vi "myRIO_BRig_Host_comm_hostRoot.vi"() -> (2 "output_hostRoot":string="C:\\BehaviorRig")   [LabVIEW 2014]
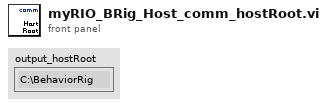
[diagram p1: front panel]
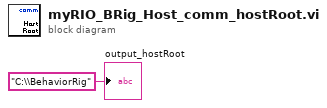
[diagram p0: block diagram]
diagram:
  "output_hostRoot" <- "C:\\BehaviorRig"
